vi "XboxControl.vi"() -> ()   [LabVIEW 2012]
uses:
  <vilib>/Utility/inputDevices.llb/closeJoystick.vi
  <vilib>/Utility/inputDevices.llb/joystickAcquire.vi
panel:
  out "joystick info":T1(array[cluster])
  in  "stop":bool
  out "X axis 1":sgl(slide) scale=-1.0..1.0
  out "Y axis 1":sgl(slide) scale=-1.0..1.0
  out "X axis 2":sgl(slide) scale=-1.0..1.0
  out "Y axis 2":sgl(slide) scale=-1.0..1.0
  out "Triggers":sgl(slide) scale=-1.0..1.0
  out "button info":T2
  out "pov 1":i32
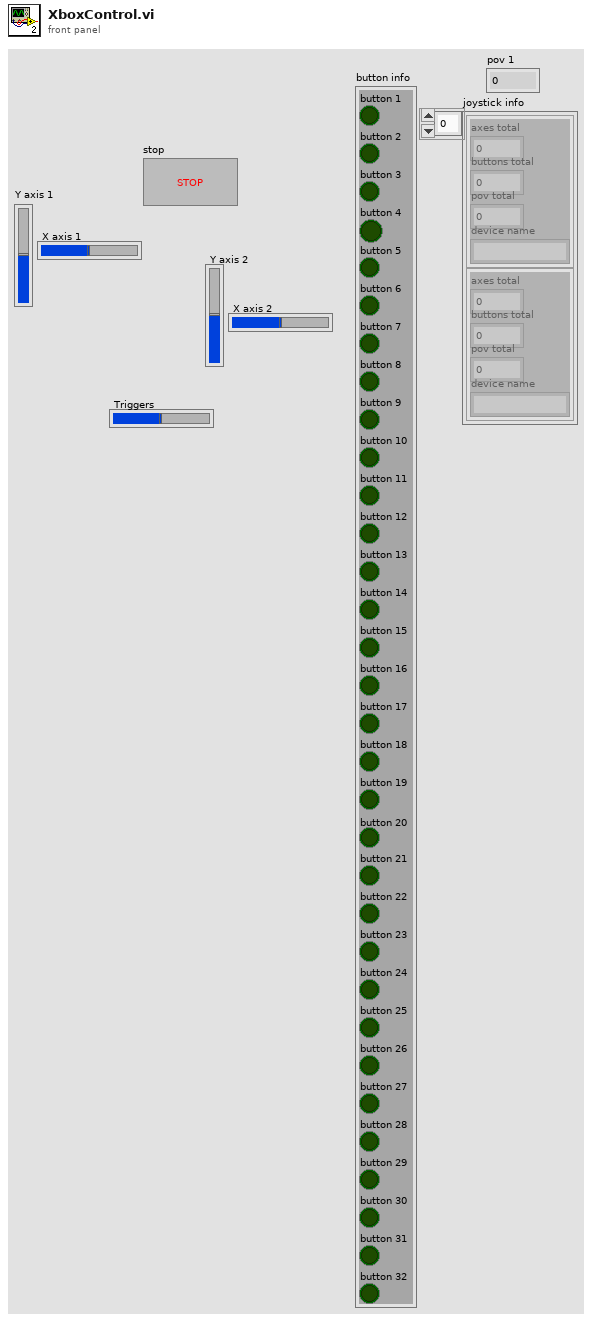
[diagram p1: front panel]
types:
  T1 = cluster{"axes total":u32, "buttons total":u32, "pov total":u32, "device name":string}[]
  T2 = cluster{"button 1":bool, "button 2":bool, "button 3":bool, "button 4":bool, "button 5":bool, "button 6":bool, "button 7":bool, "button 8":bool, "button 9":bool, "button 10":bool, "button 11":bool, "button 12":bool, "button 13":bool, "button 14":bool, "button 15":bool, "button 16":bool, "button 17":bool, "button 18":bool, "button 19":bool, "button 20":bool, "button 21":bool, "button 22":bool, "button 23":bool, "button 24":bool, "button 25":bool, "button 26":bool, "button 27":bool, "button 28":bool, "button 29":bool, "button 30":bool, "button 31":bool, "button 32":bool}
  T3 = cluster{"X axis":i32, "Y axis":i32, "Z axis":i32, "X axis rotation":i32, "Y axis rotation":i32, "Z axis rotation":i32, "U axis":i32, "V axis":i32}
  T4 = cluster{"pov 1":i32, "pov 2":i32, "pov 3":i32, "pov 4":i32}
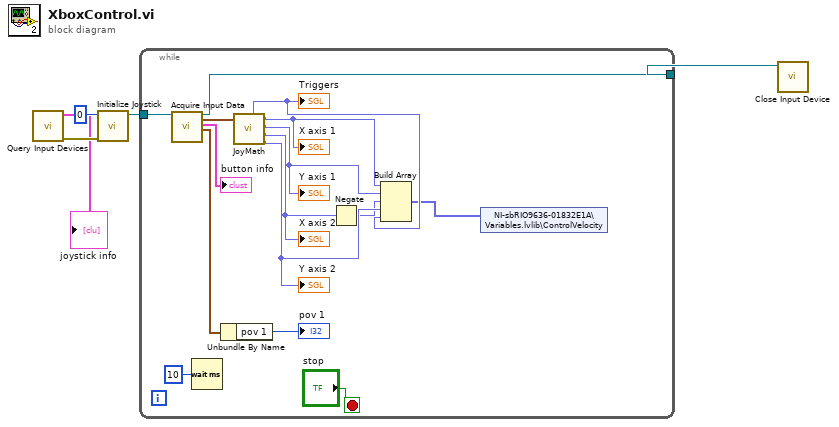
[diagram p0: block diagram]
diagram:
  n1 = call <vilib>:"Query Input Devices.vi"() -> ("error out"=w5:errorcluster, "joystick info"=→"joystick info":T1)  [unwired: 1 in, 9 out]
  n2 = call <vilib>:"Initialize Joystick.vi"("error in (no error)"=w5, "device index"=0) -> ("device ID"=w3:refnum<k1>)  [unwired: 9 out]
  n3 = while {
    tunnel: w3 -> [w20]
    tunnel: [w18] -> w2
    stop <- "stop" stop-if-true
    n4 = call-poly <vilib>:"Acquire Input Data.vi"("device ID"=w20) -> ("device ID"=w18:refnum<k1>, "axis info"=w14:T3, "button info"=→"button info":T2, "direction info"=w16:T4)  [unwired: 1 in, 14 out]
    n5 = Wait (ms)(milliseconds to wait=u32 10) -> ()  [unwired: 1 out]
    n6 = Unbundle By Name(w16) -> ("pov 1"=→"pov 1":i32)
    n7 = call "JoyMath.vi"("input cluster"=w14) -> ("Y axis 2"=w10:fxp<+/-,9,2>, "X axis 2"=w11:fxp<+/-,9,2>, "Y axis 1"=w12:fxp<+/-,9,2>, "X axis 1"=w13:fxp<+/-,9,2>, "Triggers"=w9:fxp<+/-,9,2>)  [unwired: 6 in]
    "X axis 1" <- w13
    "Y axis 1" <- w12
    "X axis 2" <- w11
    "Y axis 2" <- w10
    "Triggers" <- w9
    n8 = Negate(x=w11) -> (-x=w6:fxp<+/-,10,3>)
    n9 = Build Array(w13, w12, w6, w10, w9) -> (w8:fxp<+/-,10,3>[])
    n10 = shared-variable "NI-sbRIO9636-01832E1A\\Variables.lvlib\\ControlVelocity"(w8) -> ()  [unwired: 1 in, 1 out]
  }
  n11 = call-poly <vilib>:"Close Input Device.vi"("device ID"=w2) -> ()  [unwired: 1 in, 9 out]
